vi "SW_get_config_for_Start_Stop_pulses.vi"(0 "Sync parameters cluster input":T2={"SYNC configuration"=12, "IO 1 configuration"=1, "IO 2 configuration"=1, "IO 3 configuration"=0, "IO 4 configuration"=0, "Activate ext. RS-232"=0, "IO inversion config."=0}) -> (1 "Start/Stop out pulses config":u32, 2 "Start/Stop in config":u32, 3 "Start/Stop in config bin":bool[](array[boolean]), 4 "Start/Stop out pulses config bin":bool[](array[boolean]))   [LabVIEW 2018, in "Tracker.lvlib"]
uses:
  <vilib>/Utility/miscctls.llb/LVPointTypeDef.ctl
  Tracker.lvlib
panel:
  out "IO status indicator":T1
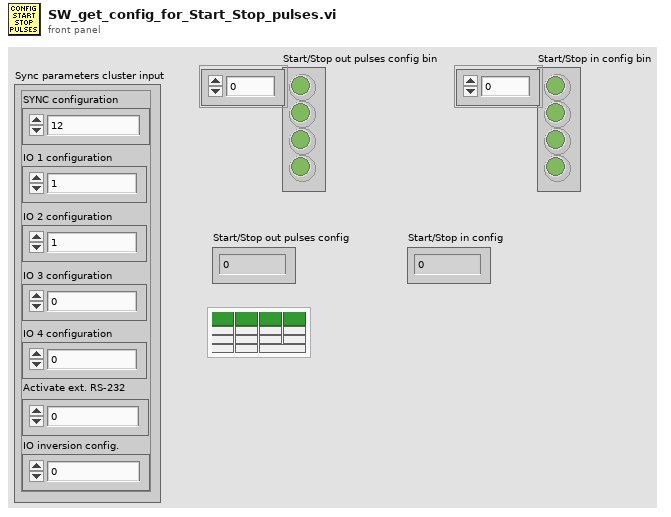
[diagram p1: front panel]
types:
  T1 = cluster{"IO1":bool, "IO2":bool, "IO3":bool, "IO4":bool, "Z1":bool, "Z2":bool, "Z3":bool, "Z4":bool, "St1":bool, "St2":bool, "St3":bool, "St4":bool, "Syn1":bool, "Syn2":bool, "RS-232 ext. activated":bool}
  T2 = cluster{"SYNC configuration":u16, "IO 1 configuration":u16, "IO 2 configuration":u16, "IO 3 configuration":u16, "IO 4 configuration":u16, "Activate ext. RS-232":u16, "IO inversion config.":u16}
  T3 = typedef "LVPointTypeDef.ctl" = cluster{"Horizontal":i16, "Vertical":i16}
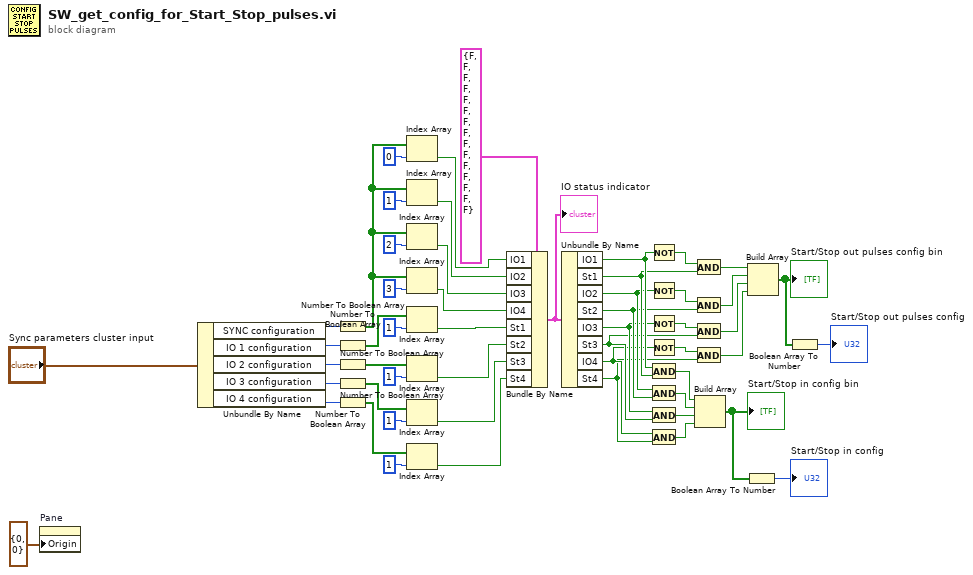
[diagram p0: block diagram]
diagram:
  n1 = property on="Pane" class="Pane"("Origin"=T3 {"Horizontal"=0, "Vertical"=0}) -> ()  [unwired: 2 in, 2 out]
  n2 = Unbundle By Name("Sync parameters cluster input") -> ("SYNC configuration"=w49:u16, "IO 1 configuration"=w43:u16, "IO 2 configuration"=w38:u16, "IO 3 configuration"=w35:u16, "IO 4 configuration"=w34:u16)
  n3 = Number To Boolean Array(number=w49) -> (Boolean array=w48:bool[])
  n4 = Number To Boolean Array(number=w43) -> (Boolean array=w42:bool[])
  n5 = Number To Boolean Array(number=w38) -> (Boolean array=w39:bool[])
  n6 = Number To Boolean Array(number=w35) -> (Boolean array=w37:bool[])
  n7 = Number To Boolean Array(number=w34) -> (Boolean array=w36:bool[])
  n8 = Index Array(array=w48, index=0) -> (element=w53:bool)
  n9 = Index Array(array=w48, index=1) -> (element=w52:bool)
  n10 = Index Array(array=w48, index=2) -> (element=w51:bool)
  n11 = Index Array(array=w48, index=3) -> (element=w50:bool)
  n12 = Index Array(array=w42, index=1) -> (element=w29:bool)
  n13 = Index Array(array=w39, index=1) -> (element=w28:bool)
  n14 = Index Array(array=w37, index=1) -> (element=w27:bool)
  n15 = Index Array(array=w36, index=1) -> (element=w26:bool)
  n16 = Bundle By Name(cluster=T1 {"IO1"=FALSE, "IO2"=FALSE, "IO3"=FALSE, "IO4"=FALSE, "Z1"=FALSE, "Z2"=FALSE, "Z3"=FALSE, "Z4"=FALSE, "St1"=FALSE, "St2"=FALSE, "St3"=FALSE, "St4"=FALSE, "Syn1"=FALSE, "Syn2"=FALSE, "RS-232 ext. activated"=FALSE} ("IO status indicator 2"), "IO1"=w53, "IO2"=w52, "IO3"=w51, "IO4"=w50, "St1"=w29, "St2"=w28, "St3"=w27, "St4"=w26) -> (w17:T1)
  "IO status indicator" <- w17
  n17 = Unbundle By Name(w17) -> ("IO1"=w8:bool, "St1"=w7:bool, "IO2"=w6:bool, "St2"=w5:bool, "IO3"=w4:bool, "St3"=w3:bool, "IO4"=w2:bool, "St4"=w1:bool)
  n18 = Not(x=w8) -> (.not. x?=w25:bool)
  n19 = Not(x=w6) -> (.not. x?=w24:bool)
  n20 = Not(x=w4) -> (.not. x?=w23:bool)
  n21 = Not(x=w2) -> (.not. x?=w22:bool)
  n22 = And(x=w8, y=w7) -> (x .and. y?=w9:bool)
  n23 = And(x=w6, y=w5) -> (x .and. y?=w10:bool)
  n24 = And(x=w4, y=w3) -> (x .and. y?=w11:bool)
  n25 = And(x=w2, y=w1) -> (x .and. y?=w12:bool)
  n26 = And(x=w25, y=w7) -> (x .and. y?=w21:bool)
  n27 = And(x=w24, y=w5) -> (x .and. y?=w20:bool)
  n28 = And(x=w23, y=w3) -> (x .and. y?=w19:bool)
  n29 = And(x=w22, y=w1) -> (x .and. y?=w18:bool)
  n30 = Build Array(w9, w10, w11, w12) -> (w13:bool[])
  "Start/Stop in config bin" <- w13
  n31 = Boolean Array To Number(Boolean array=w13) -> (number=→"Start/Stop in config":u32)
  n32 = Build Array(w21, w20, w19, w18) -> (w16:bool[])
  "Start/Stop out pulses config bin" <- w16
  n33 = Boolean Array To Number(Boolean array=w16) -> (number=→"Start/Stop out pulses config":u32)
